vi "Launch TCP data clients.vi"(9 "TCPDevDataStopQueueName":string="TCPDevStatusStopQueue", 10 "DevicetcpDataqueueName":string="DevicetcpDataqueue", 11 "TCP subscriptions info":T2) -> (1 "tcp data event":T1, 2 "StopQueue":refnum<queue>, 3 "DataQueue":refnum<queue>)   [LabVIEW 2020]
uses:
  Shared/GUI_Template/TCP subscription info cluster.ctl
  Shared/GUI_Template/GUI_master/tcp_new_data_event.ctl
  Shared/GUI_Template/GUI_master/tcp new data cluster.ctl
  Shared/MySQL/Preset Query Enum.ctl
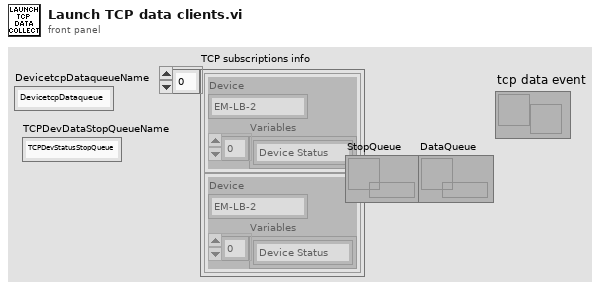
[diagram p1: front panel]
types:
  T1 = typedef "tcp_new_data_event.ctl" = refnum<user-event>
  T2 = typedef "TCP subscription info cluster.ctl" = cluster{"Device":string, "Variables":string[]}[]
  T3 = typedef "Preset Query Enum.ctl" = enum16{"Get Locations", "Get all IPs and MACs", "Get classes", "Get expt variables to set at scanstart for particular device", "Get expt devices and variables with start values", "Get expt devices and variables (with data to get)", "Get expt devices with data to get", "Get Expt devices and GUIs", "Get all devices basic properties", "Get Virtual Devices Core Info", "Get Expt names", "Get experiment basic properties", "Get experiment alarm variables", "Get MC Ports", "Get device network comm port", "Get devicetype lvclass path", "Get basic device properties", "Get Init Order", "Get all setable variables of a device", "Get device variable aliases", "Get force values of all settable variables", "Get all variables of a devicetype", "Get all variables of a device", "Get plotter details", "Get Saved Scans", "Get Scan Info", "GetGeneralGUIs", "Get expt for plotter", "Get plotter IDs from expt", "Get all devices", "Get all Virtual Devices", "Get all aliases", "Get variable and device info for Virtual Device", "GetItemLocatorIP", "Get IPs for GUIs", "Get DeviceType from Device", "GetLocalPortRange", "GetDevicePresetVariables", "Get Device Configuration", "GetAllPresetNames", "GetAllConfigurationNames", "GetPresetDeviceNames", "GetDeviceAliases", "GetDevicesOfClass"}
  T4 = typedef "tcp new data cluster.ctl" = cluster{"EventEnum":enum16{"new data", "connection status update"}, "Device name":string}
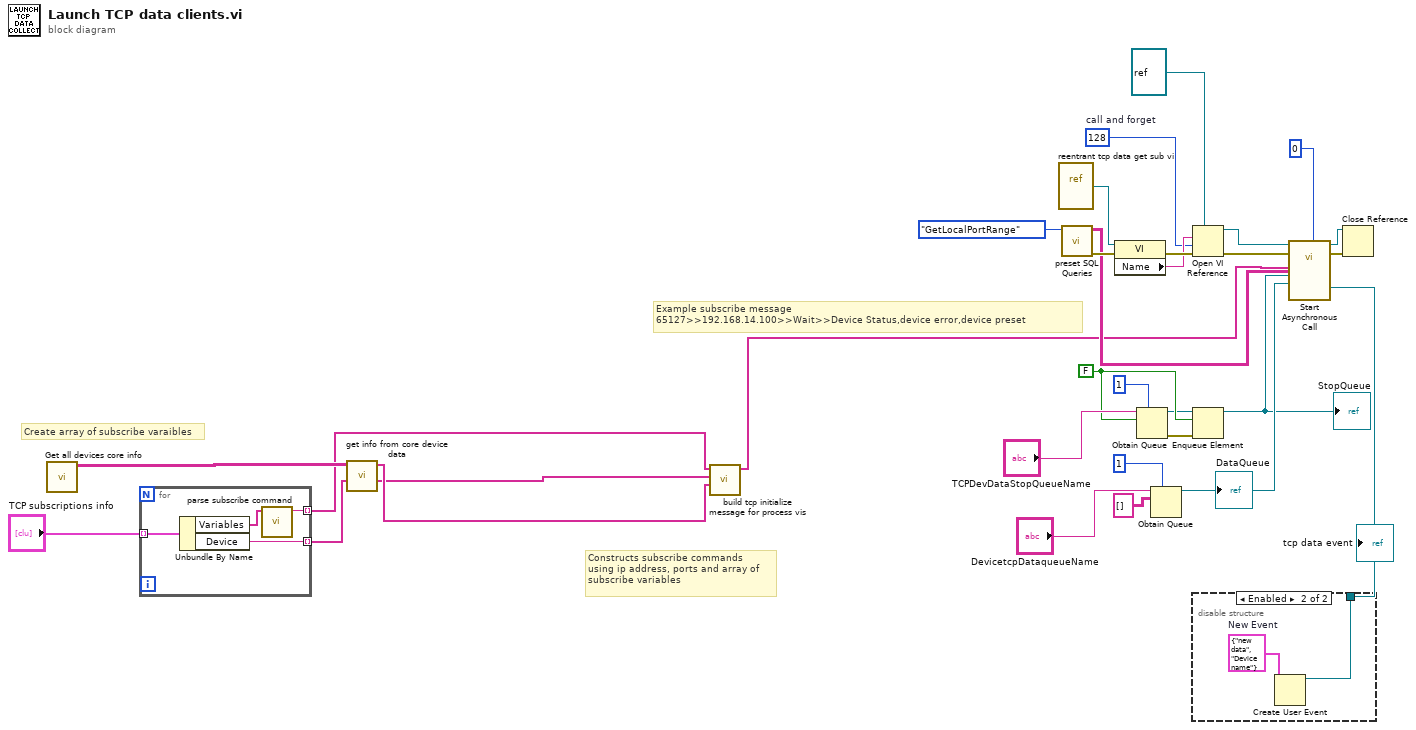
[diagram p0: block diagram]
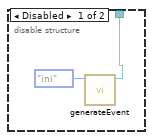
[diagram p2: hidden frame]
diagram:
  w27 = FALSE
  w9 = 128  # call and forget
  # "Constructs subscribe commands\nusing ip address, ports and array of \nsubscribe variables"
  # "Create array of subscribe varaibles"
  # "Example subscribe message\n65127>>192.168.14.100>>Wait>>Device Status,device error,device preset"
  n1 = call "Get all devices core info.vi"() -> ("> Name, devtype, ip, dev comm port, class, location for all devices>"=w6:string[][])  [unwired: 8 in, 3 out]
  n2 = for {
    tunnel: "TCP subscriptions info" -> [w35] mode=indexing
    tunnel: [w34] -> w3 mode=indexing
    tunnel: [w32] -> w2 mode=indexing
    n3 = Unbundle By Name(w35) -> ("Variables"=w33:string[], "Device"=w34:string)
    n4 = call "parse subscribe command.vi"("variable names"=w33) -> ("Subscribe command"=w32:string)  [unwired: 6 in]
  }
  n5 = call "get info from core device data.vi"("devices to get data from"=w3, "All Devices Core Info"=w6) -> ("Ports"=w7:string[], "IP Addresses"=w8:string[])  [unwired: 2 in, 2 out]
  n6 = call "build tcp initialize message for process vis.vi"("IP Addresses"=w8, "Ports"=w7, "Subscribe commands"=w2) -> ("subscribe messages\nfor process vis"=w5:string[])  [unwired: 8 in]
  n7 = vi-ref "reentrant tcp data get sub vi.vi"() -> (w17:refnum<vi>)
  n8 = call "preset SQL Queries.vi"("Preset Query"=Preset_Query_Enum."GetLocalPortRange") -> ("error out"=w21:errorcluster, "data"=w20:string[][])  [unwired: 8 in, 1 out]
  n9 = property class="VI"(reference=w17, error in=w21) -> (error out=w16:errorcluster, "Name"=w15:string)  [unwired: 1 out]
  n10 = Obtain Queue(max queue size (-1, unlimited)=1, name (unnamed)="TCPDevDataStopQueueName", element data type=w27) -> (queue out=w25:refnum<queue>, error out=w26:errorcluster)  [unwired: 2 in, 1 out]
  n11 = Obtain Queue(max queue size (-1, unlimited)=1, name (unnamed)="DevicetcpDataqueueName", element data type=string[][] [] ("Data in")) -> (queue out=w31:refnum<queue>)  [unwired: 2 in, 2 out]
  "DataQueue" <- w31
  n12 = Open VI Reference(type specifier VI Refnum (for type only)=refnum<vi> refnum, vi path=w15, options=w9, error in (no error)=w16) -> (vi reference=w11:refnum<vi>, error out=w12:errorcluster)  [unwired: 2 in]
  n13 = Enqueue Element(queue=w25, element=w27, error in (no error)=w26) -> (queue out=w30:refnum<queue>)  [unwired: 1 in, 2 out]
  "StopQueue" <- w30
  n14 = disable-structure shown="Enabled" {
    disable-tunnel: [w36 w38] -> w1
    frame Disabled {
      n15 = call "generateEvent.vi"("command"=enum16{"ini", "get", "close"}."ini") -> ("tcp data event"=w36:T1)  [unwired: 9 in, 1 out]
    }
    frame Enabled {
      w39 = T4 {"EventEnum"=enum."new data", "Device name"="Device name"}  # New Event
      n16 = Create User Event(user event datatype=w39) -> (user event=w38:refnum<user-event>)  [unwired: 1 in, 1 out]
    }
  }
  "tcp data event" <- w1
  n17 = call-by-ref "Start Asynchronous Call"(reference=w11, error in=w12, "ms to wait"=u32 0, "tcp data event"=w1, "Ports"=w20, "tcpDataqueue"=w31, "Stopqueue"=w30, "subscribe messages for process vis"=w5) -> (reference out=w14:refnum<vi>, error out=w13:errorcluster)  [unwired: 5 in, 1 out]
  n18 = Close Reference(reference=w14, error in (no error)=w13) -> ()  [unwired: 1 out]
